vi "devref data base FG.vi"(9 "DevRef to Get":T11, 11 "Menu":T12) -> (0 "error out":errorcluster, 1 "Selected Sensor":T5, 2 "Selected Encoder":T1={"DevStatus"={"status"=FALSE, "code"=0, "source"=""}, "EncoderIndex"=enum."Invalid", "CounterIndex"=enum."Invalid", "DistancePerCount"=1.0, "Decoding Type"=enum."4x"}, 3 "Selected Solenoid":T8={"DevStatus"={"status"=FALSE, "code"=0, "source"=""}, "Solenoid Module"=enum."Solenoid Module 1", "Forward Solenoid Channel"=enum."Invalid", "Reverse Solenoid Channel"=enum."Invalid"}, 5 "right drive encoder":T1={"DevStatus"={"status"=FALSE, "code"=0, "source"=""}, "EncoderIndex"=enum."Invalid", "CounterIndex"=enum."Invalid", "DistancePerCount"=1.0, "Decoding Type"=enum."4x"}, 7 "left drive encoder":T1={"DevStatus"={"status"=FALSE, "code"=0, "source"=""}, "EncoderIndex"=enum."Invalid", "CounterIndex"=enum."Invalid", "DistancePerCount"=1.0, "Decoding Type"=enum."4x"})   [LabVIEW 2013]
uses:
  typedefs/fg_getset.ctl
  typedefs/devref to get.ctl
  <vilib>/Rock Robotics/WPI/Solenoid/WPI_SolenoidDevRef.ctl
  <vilib>/Rock Robotics/SystemInterfaces/Typedef/FPGA_TypedefSolenoidModule.ctl
  <vilib>/Rock Robotics/WPI/Solenoid/WPI_SolenoidChannel.ctl
  <vilib>/Rock Robotics/WPI/DigitalInput/WPI_DigitalInputDevRef.ctl
  <vilib>/Rock Robotics/SystemInterfaces/DIO/FPGA_DIOChannel.ctl
  <vilib>/Rock Robotics/SystemInterfaces/Typedef/FPGA_TypedefDigitalModule.ctl
  <vilib>/Rock Robotics/WPI/Encoder/WPI_EncoderDevRef.ctl
  <vilib>/Rock Robotics/SystemInterfaces/Encoder/FPGA_EncoderIdx.ctl
  <vilib>/Rock Robotics/SystemInterfaces/Counter/FPGA_CounterCtrSystemIndex.ctl
  <vilib>/Rock Robotics/WPI/Encoder/WPI_EncoderType.ctl
panel:
  # "A Functional Global that stores refnums for \ncommonly used devices \nso as to not need to get them repeatedly"
  # "it is only set once"
  # "Option to Select Also..."
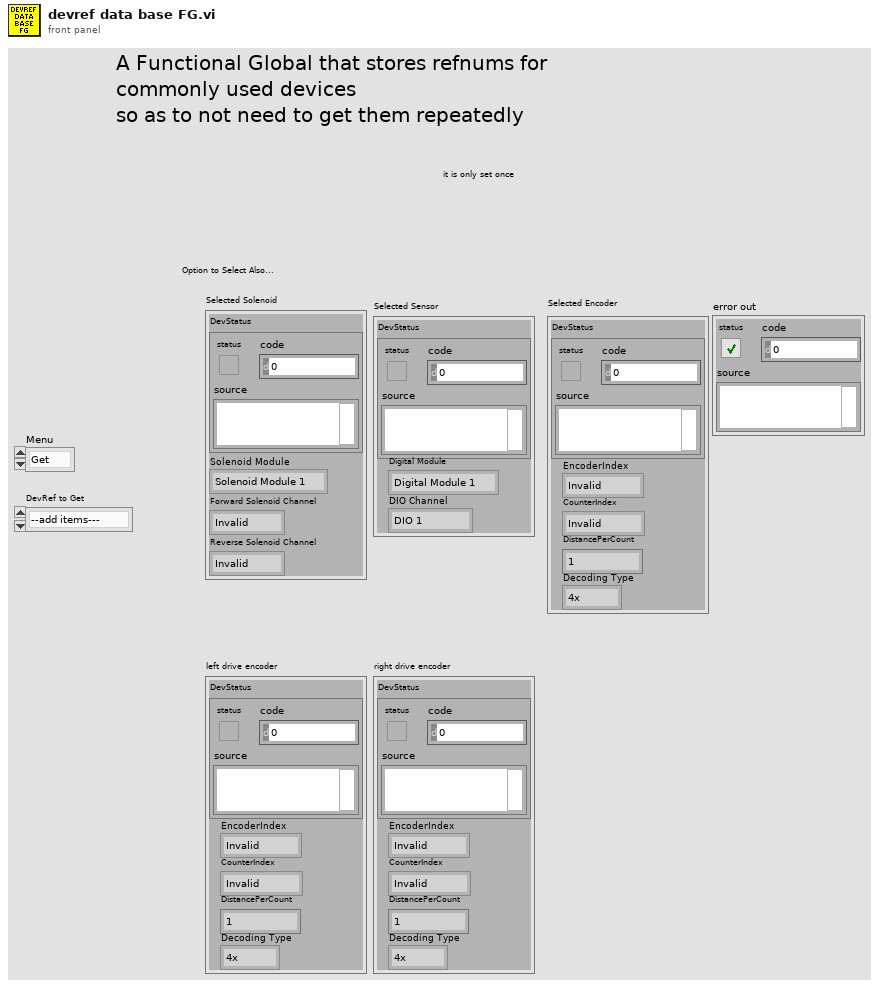
[diagram p1: front panel]
types:
  T1 = typedef "WPI_EncoderDevRef.ctl" = cluster{"DevStatus":errorcluster, "EncoderIndex":T2, "CounterIndex":T3, "DistancePerCount":dbl, "Decoding Type":T4}
  T2 = typedef "FPGA_EncoderIdx.ctl" = enum8{"Enc 0", "Enc 1", "Enc 2", "Enc 3", "Invalid"}
  T3 = typedef "FPGA_CounterCtrSystemIndex.ctl" = enum8{"Ctr 0", "Ctr 1", "Ctr 2", "Ctr 3", "Ctr 4", "Ctr 5", "Ctr 6", "Ctr 7", "Invalid"}
  T4 = typedef "WPI_EncoderType.ctl" = enum16{"1x", "2x", "4x"}
  T5 = typedef "WPI_DigitalInputDevRef.ctl" = cluster{"DevStatus":errorcluster, "DIO Channel":T6, "Digital Module":T7}
  T6 = typedef "FPGA_DIOChannel.ctl" = enum8{"DIO 1", "DIO 2", "DIO 3", "DIO 4", "DIO 5", "DIO 6", "DIO 7", "DIO 8", "DIO 9", "DIO 10", "DIO 11", "DIO 12", "DIO 13", "DIO 14", "Invalid"}
  T7 = typedef "FPGA_TypedefDigitalModule.ctl" = enum16{"Digital Module 1", "Digital Module 2"}
  T8 = typedef "WPI_SolenoidDevRef.ctl" = cluster{"DevStatus":errorcluster, "Solenoid Module":T9, "Forward Solenoid Channel":T10, "Reverse Solenoid Channel":T10}
  T9 = typedef "FPGA_TypedefSolenoidModule.ctl" = enum16{"Solenoid Module 1", "Solenoid Module 2"}
  T10 = typedef "WPI_SolenoidChannel.ctl" = enum8{"Solenoid 1", "Solenoid 2", "Solenoid 3", "Solenoid 4", "Solenoid 5", "Solenoid 6", "Solenoid 7", "Solenoid 8", "Invalid"}
  T11 = typedef "devref to get.ctl" = enum16{"--add items---"}
  T12 = typedef "fg_getset.ctl" = enum16{"Get", "Set"}
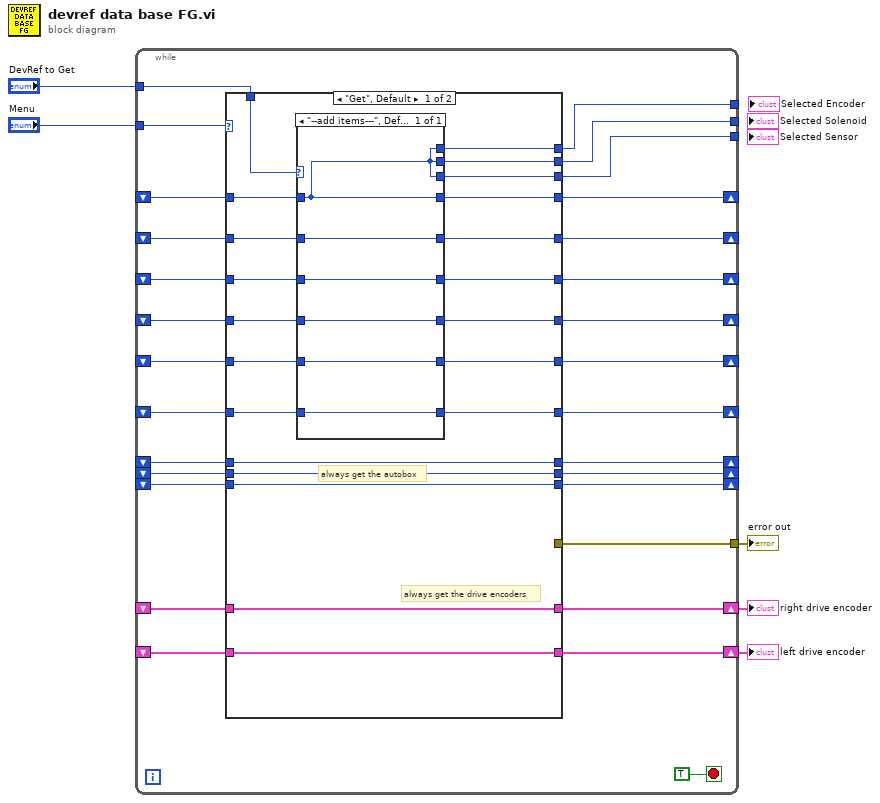
[diagram p0: block diagram]
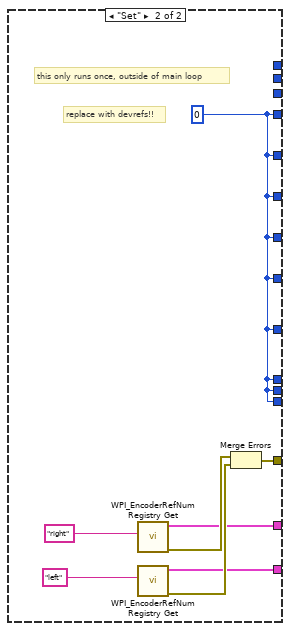
[diagram p2: hidden frame]
diagram:
  n1 = while {
    shift-right: [w28] -> _
    shift-left: _ -> [w33]
    shift-right: [w27] -> _
    shift-left: _ -> [w32]
    shift-right: [w26] -> _
    shift-left: _ -> [w30]
    shift-right: [w25] -> _
    shift-left: _ -> [w29]
    tunnel: "Menu" -> [w31]
    shift-right: [w23] -> _
    shift-left: _ -> [w24]
    tunnel: "DevRef to Get" -> [w22]
    tunnel: [w21] -> _
    tunnel: [w20] -> _
    shift-right: [w18] -> _
    shift-left: _ -> [w19]
    tunnel: [w17] -> _
    shift-right: [w16] -> _
    shift-left: _ -> [w15]
    shift-right: [w14] -> w2
    shift-left: _ -> [w11]
    shift-right: [w13] -> w1
    shift-left: _ -> [w10]
    tunnel: [w12] -> w3
    shift-right: [w9] -> _
    shift-left: _ -> [w7]
    shift-right: [w8] -> _
    shift-left: _ -> [w6]
    stop <- TRUE stop-if-true
    n2 = case shown="\"Get\", Default" w31 {
      tunnel: w33 -> [w54 _]
      tunnel: w32 -> [w53 _]
      tunnel: w30 -> [w52 _]
      tunnel: w29 -> [w51 _]
      tunnel: [w43 w62] -> w28
      tunnel: [w44 w62] -> w27
      tunnel: [w45 w62] -> w26
      tunnel: [w46 w62] -> w25
      tunnel: w24 -> [w50 _]
      tunnel: [w47 w62] -> w23
      tunnel: w22 -> [w55 _]
      tunnel: [w49 _] -> w21
      tunnel: [w48 _] -> w20
      tunnel: w19 -> [w42 _]
      tunnel: [w41 w62] -> w18
      tunnel: [w40 _] -> w17
      tunnel: [w37 w62] -> w16
      tunnel: w15 -> [w37 _]
      tunnel: [w39 w65] -> w14
      tunnel: [w38 w64] -> w13
      tunnel: [_ w63] -> w12
      tunnel: w11 -> [w39 _]
      tunnel: w10 -> [w38 _]
      tunnel: [w36 w62] -> w9
      tunnel: [w35 w62] -> w8
      tunnel: w7 -> [w36 _]
      tunnel: w6 -> [w35 _]
      frame "Get", Default {
        # "always get the autobox"
        # "always get the drive encoders"
        n3 = case shown="\"--add items---\", Default" w55 {
          tunnel: w54 -> [w56]
          tunnel: w53 -> [w58]
          tunnel: w52 -> [w59]
          tunnel: w51 -> [w60]
          tunnel: w50 -> [w61]
          tunnel: [w56] -> w49
          tunnel: [w56] -> w48
          tunnel: [w61] -> w47
          tunnel: [w60] -> w46
          tunnel: [w59] -> w45
          tunnel: [w58] -> w44
          tunnel: [w56] -> w43
          tunnel: w42 -> [w57]
          tunnel: [w57] -> w41
          tunnel: [w56] -> w40
          frame "--add items---", Default {
          }
        }
      }
      frame "Set" {
        w62 = 0
        # "replace with devrefs!!"
        # "this only runs once, outside of main loop"
        n4 = call <vilib>:"WPI_EncoderRefNum Registry Get.vi"("refnum name"="right") -> ("error out"=w67:errorcluster, "EncoderDevRef"=w65:T1)  [unwired: 9 in]
        n5 = call <vilib>:"WPI_EncoderRefNum Registry Get.vi"("refnum name"="left") -> ("error out"=w66:errorcluster, "EncoderDevRef"=w64:T1)  [unwired: 9 in]
        n6 = Merge Errors(w67, w66) -> (w63:errorcluster)
      }
    }
  }
  "error out" <- w3
  "right drive encoder" <- w2
  "left drive encoder" <- w1
